vi "Gaussian surface with rotation and offset model3.vi"(3 "output control":T1, 4 "data":variant, 5 "X":dbl[](array[numeric]), 6 "a":dbl[](array[numeric])) -> (0 "error out":errorcluster, 1 "f'(X,a)":dbl[][](array[numeric]), 2 "f(X,a)":dbl[](array[numeric]))   [LabVIEW 2015]
doc: "Gaussian surface with offset model"
uses:
  <vilib>/gmath/NumericalOptimization/LM_output select.ctl
  <vilib>/gmath/NI_Gmath.lvlib
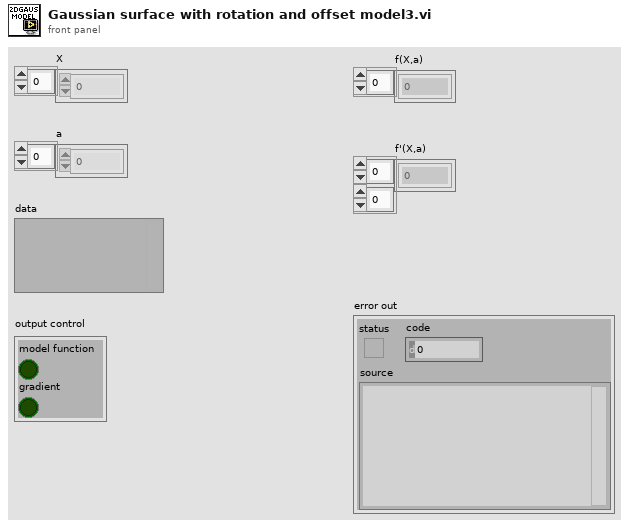
[diagram p1: front panel]
types:
  T1 = typedef "NI_Gmath.lvlib/LM_output select.ctl" = cluster{"model function":bool, "gradient":bool}
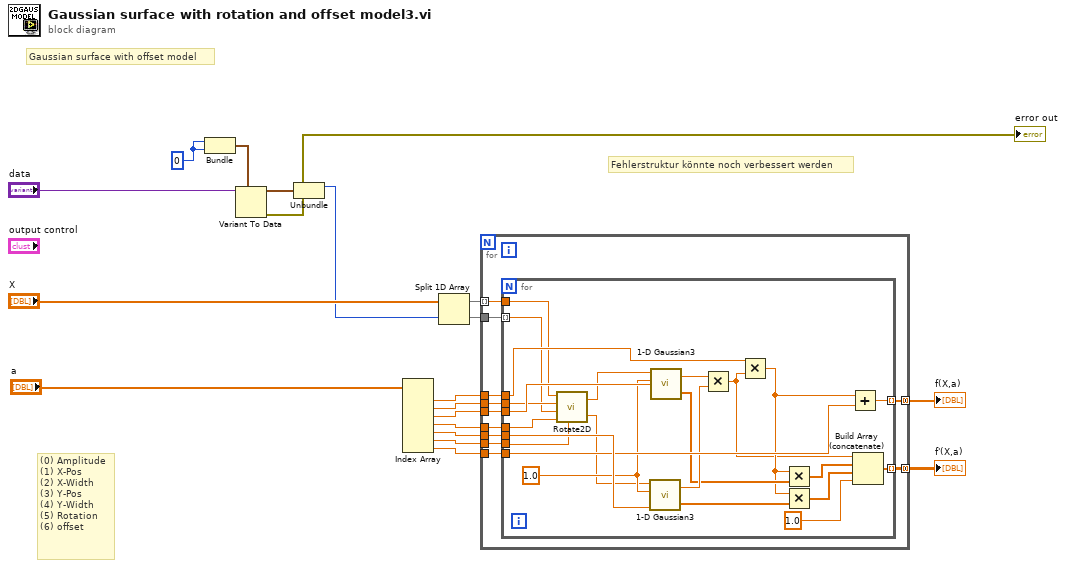
[diagram p0: block diagram]
diagram:
  w14 = 0
  # "(0) Amplitude\n(1) X-Pos\n(2) X-Width\n(3) Y-Pos\n(4) Y-Width\n(5) Rotation\n(6) offset"
  # "Fehlerstruktur könnte noch verbessert werden"
  # "Gaussian surface with offset model"
  n1 = Bundle(w14, w14) -> (w9:cluster{i32, i32})  [unwired: 1 out]
  n2 = Variant To Data(type=w9, Variant="data") -> (data=w5:cluster{i32, i32}, error out=→"error out":errorcluster)  [unwired: 1 in]
  n3 = Unbundle(w5) -> (w4:i32)  [unwired: 1 out]
  n4 = Index Array(array="a") -> (element #1=w19:dbl, element #2=w18:dbl, element #3=w17:dbl, element #4=w11:dbl, element #5=w10:dbl, element #6=w1:dbl, element #7=w2:dbl)  [unwired: 7 in]
  n5 = Split 1D Array(array="X", index=w4) -> (first subarray=w13:dbl[], second subarray=w12:dbl[])
  n6 = for {
    tunnel: w19 -> [w30]
    tunnel: w18 -> [w29]
    tunnel: w17 -> [w28]
    tunnel: w11 -> [w25]
    tunnel: w10 -> [w24]
    tunnel: w2 -> [w23]
    tunnel: w13 -> [w27] mode=indexing
    tunnel: w12 -> [w26]
    tunnel: [w22] -> w7 mode=concatenating
    tunnel: [w21] -> w6 mode=concatenating
    tunnel: w1 -> [w20]
    n7 = for {
      tunnel: [w52] -> w22 mode=indexing
      tunnel: w30 -> [w53]
      tunnel: w29 -> [w36]
      tunnel: w28 -> [w51]
      tunnel: w27 -> [w37]
      tunnel: w26 -> [w35] mode=indexing
      tunnel: w25 -> [w34]
      tunnel: w24 -> [w50]
      tunnel: w23 -> [w49]
      tunnel: [w45] -> w21 mode=indexing
      tunnel: w20 -> [w33]
      w48 = 1.0 ("a")
      n8 = call "Rotate2D.vi"("x"=w37, "mx"=w36, "y"=w35, "my"=w34, "alpha(rad)"=w33) -> ("xout"=w32:dbl, "yout"=w31:dbl)
      n9 = call "1-D Gaussian3.vi"("sigma"=w50, "a"=w48, "x"=w31) -> ("y'"=w42:dbl[], "y"=w46:dbl)  [unwired: 1 in]
      n10 = call "1-D Gaussian3.vi"("sigma"=w51, "a"=w48, "x"=w32) -> ("y'"=w44:dbl[], "y"=w47:dbl)  [unwired: 1 in]
      n11 = Multiply(x=w47, y=w46) -> (x*y=w38:dbl)
      n12 = Multiply(x=w53, y=w38) -> (x*y=w39:dbl)
      n13 = Multiply(x=w39, y=w44) -> (x*y=w43:dbl[])
      n14 = Multiply(x=w39, y=w42) -> (x*y=w41:dbl[])
      n15 = Add(x=w39, y=w49) -> (x+y=w52:dbl)
      n16 = Build Array (concatenate)(w38, w43, w41, 1.0) -> (w45:dbl[])
    }
  }
  "f(X,a)" <- w7
  "f'(X,a)" <- w6
